vi "Config SoftCal.vi"(0 "VISA resource name":refnum<visa-resource-name>, 1 "First Temperature Point (4.2000)":dbl=4.2 min=2.0 max=10.0 step=0.0001 format="%.4f", 2 "Second Temperature Point (77.3500)":dbl=77.35 min=50.0 max=100.0 step=0.0001 format="%.4f", 3 "Third Temperature Point (305.0000)":dbl=305.0 min=200.0 max=325.0 step=0.0001 format="%.4f", 5 "Standard Curve (1)":dbl=1.0 min=1.0 max=20.0 step=1.0, 7 "User Curve(21)":dbl=21.0 min=21.0 max=60.0 step=1.0, 9 "Serial Number (\"\")":string, 11 "error in (no error)":errorcluster, 12 "First Sensor Units Point (1.62622)":dbl=1.62622 min=1.42039 max=1.6878 step=1e-05 format="%.5f", 13 "Second Sensor Units Point (1.02032)":dbl=1.02032 min=0.9755 max=1.07051 step=1e-05 format="%.5f", 14 "Third Sensor Units Point (0.50691)":dbl=0.50691 min=0.4586 max=0.75552 step=1e-05 format="%.5f") -> (4 "VISA resource name out":refnum<visa-resource-name>, 15 "error out":errorcluster)   [LabVIEW 2024, in "Lake Shore Cryotronics 340.lvlib"]
doc: "This VI generates a softCal curve. Curves are not permanently updated in the curve FLASH until a Save Curve command has been issued using the LSCI 340 Action Save Curve to Flash.vi"
uses:
  Lake Shore Cryotronics 340.lvlib
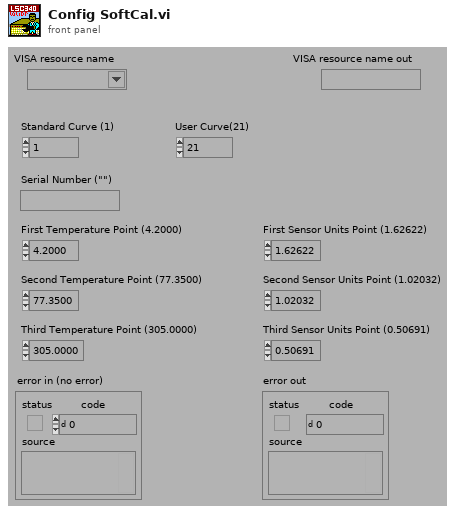
[diagram p1: front panel]
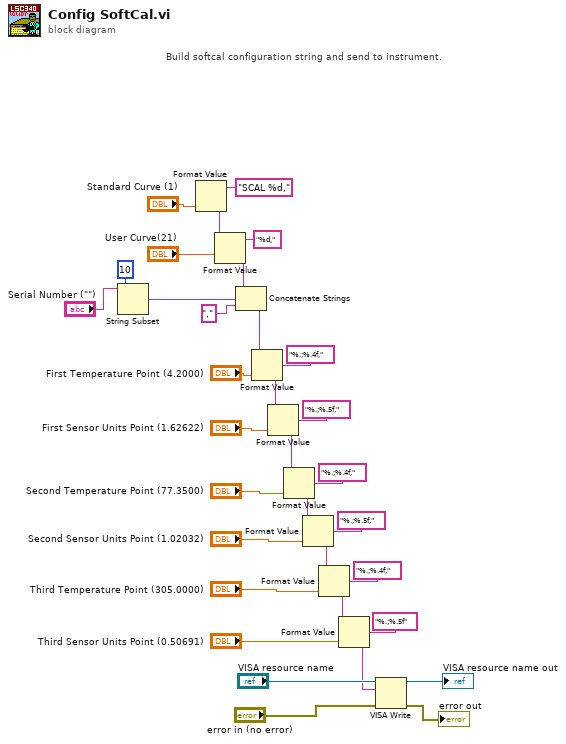
[diagram p0: block diagram]
diagram:
  # "Build softcal configuration string and send to instrument."
  n1 = String Subset(string="Serial Number (\"\")", length (rest)=10) -> (substring=w32:string)  [unwired: 1 in]
  n2 = Format Value(format string="SCAL %d,", value (0)="Standard Curve (1)") -> (output string=w25:string)  [unwired: 1 in]
  n3 = Format Value(string ("")=w25, format string="%d,", value (0)="User Curve(21)") -> (output string=w24:string)
  n4 = Concatenate Strings(w24, w32, ",") -> (w22:string)
  n5 = Format Value(string ("")=w22, format string="%.;%.4f,", value (0)="First Temperature Point (4.2000)") -> (output string=w1:string)
  n6 = Format Value(string ("")=w1, format string="%.;%.5f,", value (0)="First Sensor Units Point (1.62622)") -> (output string=w17:string)
  n7 = Format Value(string ("")=w17, format string="%.;%.4f,", value (0)="Second Temperature Point (77.3500)") -> (output string=w14:string)
  n8 = Format Value(string ("")=w14, format string="%.;%.5f,", value (0)="Second Sensor Units Point (1.02032)") -> (output string=w11:string)
  n9 = Format Value(string ("")=w11, format string="%.;%.4f,", value (0)="Third Temperature Point (305.0000)") -> (output string=w8:string)
  n10 = Format Value(string ("")=w8, format string="%.;%.5f", value (0)="Third Sensor Units Point (0.50691)") -> (output string=w2:string)
  n11 = VISA Write(VISA resource name="VISA resource name", write buffer=w2, error in (no error)="error in (no error)") -> (VISA resource name out=→"VISA resource name out":refnum<visa-resource-name>, error out=→"error out":errorcluster)  [unwired: 1 out]
